vi "SelectMenu5 1.vi"(0 "XRef":T10, 1 "Tag":T5, 2 "Point":T8, 3 "Menu Type":T7, 4 "State In":T1) -> (14 "Reply":T4, 15 "Handled?":T6, 16 "Multi Object Popup Options":T3, 17 "Fatal Error Out":T2, 18 "State Out":T1)   [LabVIEW 2013, in "VireoFunctionNode.xnode"]
uses:
  VireoFunctionNode.xnode
  <vilib>/XNodeSupport/XNodeString.ctl
  <vilib>/XNodeSupport/NI_XNodeSupport.lvlib
  <vilib>/XNodeSupport/XNodeStringArray.ctl
  <vilib>/XNodeSupport/XNodeXNodeRef.ctl
  <vilib>/XNodeSupport/XNodeInt.ctl
  <vilib>/XNodeSupport/XNodePoint.ctl
  <vilib>/XNodeSupport/XNodeMenuType.ctl
  <vilib>/XNodeSupport/XNodeBool.ctl
  <vilib>/XNodeSupport/XNodeMultiObjectPopupOptions.ctl
  <vilib>/XNodeSupport/XNodeErrorCluster.ctl
  State 1.ctl
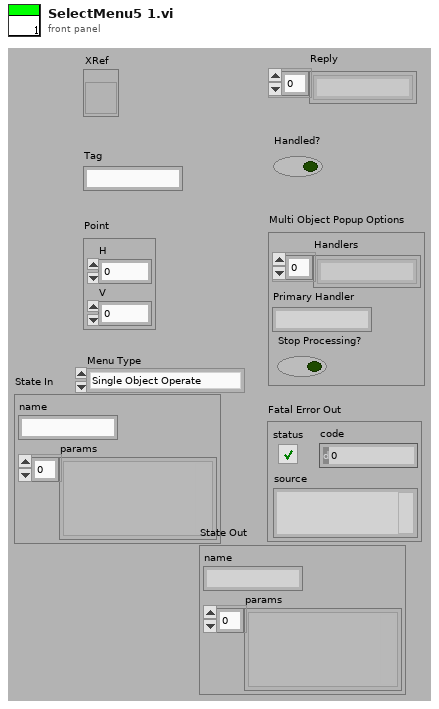
[diagram p1: front panel]
types:
  T1 = typedef "VireoFunctionNode.xnode/State 1.ctl" = cluster{"name":string, "params":variant[]}
  T2 = typedef "NI_XNodeSupport.lvlib/XNodeErrorCluster.ctl" = errorcluster
  T3 = typedef "NI_XNodeSupport.lvlib/XNodeMultiObjectPopupOptions.ctl" = cluster{"Handlers":T4, "Primary Handler":T5, "Stop Processing?":T6}
  T4 = typedef "NI_XNodeSupport.lvlib/XNodeStringArray.ctl" = T5[]
  T5 = typedef "NI_XNodeSupport.lvlib/XNodeString.ctl" = string
  T6 = typedef "NI_XNodeSupport.lvlib/XNodeBool.ctl" = bool
  T7 = typedef "NI_XNodeSupport.lvlib/XNodeMenuType.ctl" = enum32{"Single Object Operate", "Single Object Popup", "Multi Object Popup Master", "Multi Object Popup Other"}
  T8 = typedef "NI_XNodeSupport.lvlib/XNodePoint.ctl" = cluster{"H":T9, "V":T9}
  T9 = typedef "NI_XNodeSupport.lvlib/XNodeInt.ctl" = i32
  T10 = typedef "NI_XNodeSupport.lvlib/XNodeXNodeRef.ctl" = refnum<vi>
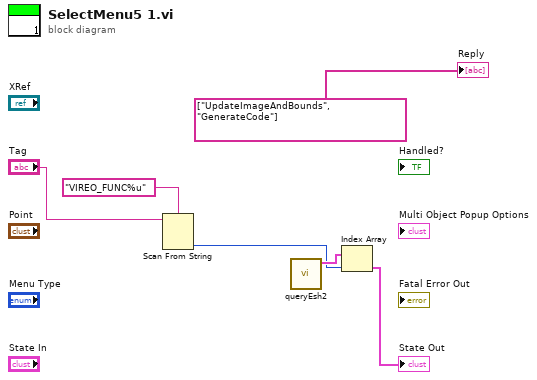
[diagram p0: block diagram]
diagram:
  n1 = Scan From String(format string="VIREO_FUNC%u", input string="Tag") -> (output 1=w3:u32)  [unwired: 3 in, 3 out]
  n2 = call "queryEsh2.vi"() -> ("Array"=w4:cluster{"name":string, "params":variant[]}[])  [unwired: 11 in]
  n3 = Index Array(array=w4, index=w3) -> (element=→"State Out":cluster{"name":string, "params":variant[]})
  "Reply" <- T4 ["UpdateImageAndBounds", "GenerateCode"] ("Reply")
